vi "Draw circle.vi"(8 "error in (no error)":errorcluster, 10 "Detail in":T1, 11 "Image in":T2) -> (0 "error out":errorcluster, 3 "Image out":T2)   [LabVIEW 2019]
uses:
  <vilib>/vision/Image Controls.llb/IMAQ Image.ctl
  <vilib>/vision/NI_Vision_Development_Module.lvlib
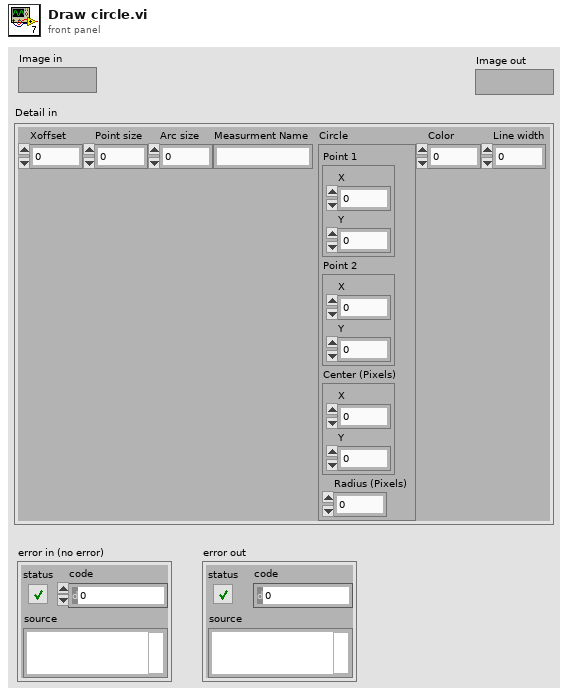
[diagram p1: front panel]
types:
  T1 = cluster{"Xoffset":i32, "Point size":dbl, "Arc size":dbl, "Measurment Name":string, "Circle":cluster{"Point 1":cluster{"X":sgl, "Y":sgl}, "Point 2":cluster{"X":sgl, "Y":sgl}, "Center (Pixels)":cluster{"X":sgl, "Y":sgl}, "Radius (Pixels)":dbl}, "Color":u32, "Line width":i32}
  T2 = typedef "IMAQ Image.ctl" = refnum<image>
  T3 = cluster{"Point 1":cluster{"X":sgl, "Y":sgl}, "Point 2":cluster{"X":sgl, "Y":sgl}, "Center (Pixels)":cluster{"X":sgl, "Y":sgl}, "Radius (Pixels)":dbl}
  T4 = cluster{"Left":i32, "Top":i32, "Right":i32, "Bottom":i32}
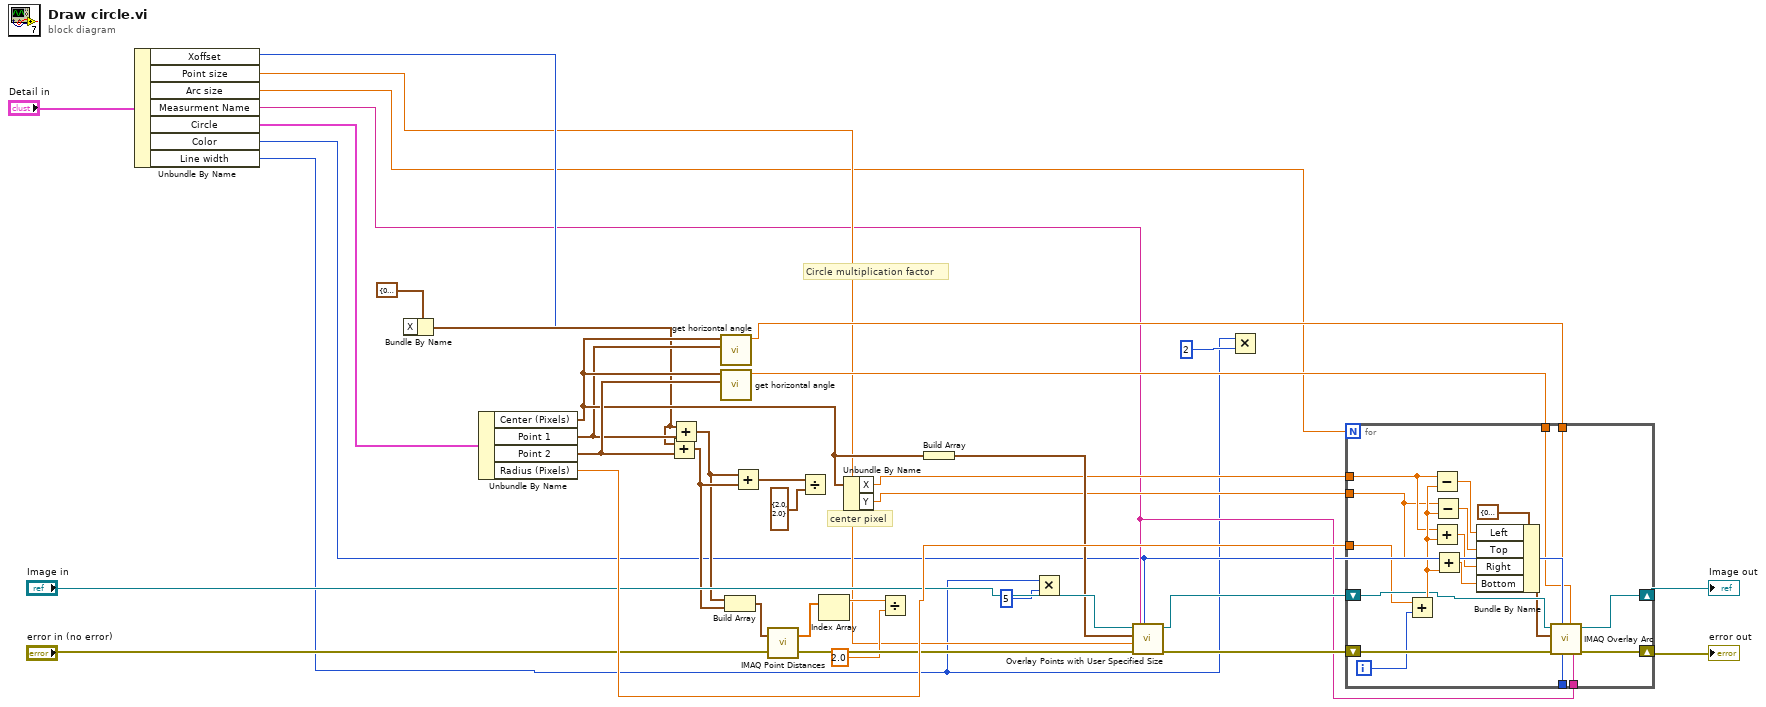
[diagram p0: block diagram]
diagram:
  # "Circle multiplication factor"
  # "center pixel"
  n1 = Unbundle By Name("Detail in") -> ("Xoffset"=w7:i32, "Point size"=w6:dbl, "Arc size"=w5:dbl, "Measurment Name"=w4:string, "Circle"=w3:T3, "Color"=w2:u32, "Line width"=w1:i32)
  n2 = Bundle By Name(cluster=cluster{"X":sgl, "Y":sgl} {"X"=0.0, "Y"=0.0} ("x"), "X"=w7) -> (w20:cluster{"X":sgl, "Y":sgl})
  n3 = Unbundle By Name(w3) -> ("Center (Pixels)"=w33:cluster{"X":sgl, "Y":sgl}, "Point 1"=w32:cluster{"X":sgl, "Y":sgl}, "Point 2"=w34:cluster{"X":sgl, "Y":sgl}, "Radius (Pixels)"=w31:dbl)
  n4 = Add(x=w20, y=w34) -> (x+y=w12:cluster{"X":sgl, "Y":sgl})
  n5 = Add(x=w20, y=w32) -> (x+y=w11:cluster{"X":sgl, "Y":sgl})
  n6 = call "get horizontal angle.vi"("Point 2"=w32, "Point 1"=w33) -> ("Angle w.r.t horizontal\n(in degrees)"=w35:sgl)  [unwired: 9 in]
  n7 = call "get horizontal angle.vi"("Point 2"=w34, "Point 1"=w33) -> ("Angle w.r.t horizontal\n(in degrees)"=w36:sgl)  [unwired: 9 in]
  n8 = Build Array(w11, w12) -> (w13:cluster{"X":sgl, "Y":sgl}[])
  n9 = Add(x=w11, y=w12) -> (x+y=w9:cluster{"X":sgl, "Y":sgl})
  n10 = call "IMAQ Point Distances"("Points"=w13, "error in (no error)"="error in (no error)") -> ("Distances"=w14:sgl[], "error out"=w26:errorcluster)  [unwired: 3 in]
  n11 = Divide(x=w9, y=cluster{"X":sgl, "Y":sgl} {"X"=2.0, "Y"=2.0}) -> ()  [unwired: 1 out]
  n12 = Index Array(array=w14) -> (element=w15:sgl)  [unwired: 1 in]
  n13 = Unbundle By Name(w33) -> ("X"=w21:sgl, "Y"=w22:sgl)
  n14 = Divide(x=w15, y=sgl 2.0) -> ()  [unwired: 1 out]
  n15 = Build Array(w33) -> (w28:cluster{"X":sgl, "Y":sgl}[])
  n16 = Multiply(x=w1, y=u32 5 ("Point Diameter (5)")) -> ()  [unwired: 1 out]
  n17 = call "Overlay Points with User Specified Size.vi"("Color"=w2, "Group"=w4, "error in"=w26, "Point Diameter (5)"=w6, "Points"=w28, "Image In"="Image in") -> ("error out"=w27:errorcluster, "Image Out"=w30:T2)  [unwired: 4 in]
  n18 = Multiply(x=w1, y=2) -> ()  [unwired: 1 out]
  n19 = for {
    N: w5 -> [_]
    shift-right: [w41] -> w18
    shift-left: w27 -> [w49]
    tunnel: w21 -> [w48]
    tunnel: w22 -> [w47]
    shift-right: [w46] -> w25
    shift-left: w30 -> [w45]
    tunnel: w31 -> [w43]
    tunnel: w2 -> [w42]
    tunnel: w35 -> [w39]
    tunnel: w36 -> [w38]
    tunnel: w4 -> [w37]
    i -> [w40]
    n20 = Add(x=w43, y=w40) -> (x+y=w50:dbl)
    n21 = Subtract(x=w48, y=w50) -> (x-y=w54:dbl)
    n22 = Add(x=w48, y=w50) -> (x+y=w52:dbl)
    n23 = Subtract(x=w47, y=w50) -> (x-y=w53:dbl)
    n24 = Add(x=w47, y=w50) -> (x+y=w51:dbl)
    n25 = Bundle By Name(cluster=T4 {"Left"=0, "Top"=0, "Right"=0, "Bottom"=0} ("Bounding Rectangle"), "Left"=w54, "Top"=w53, "Right"=w52, "Bottom"=w51) -> (w44:T4)
    n26 = call "IMAQ Overlay Arc"("Group"=w37, "End Angle (degrees)"=w38, "Color"=w42, "Start Angle (degrees)"=w39, "error in (no error)"=w49, "Bounding Rectangle"=w44, "Image"=w45) -> ("error out"=w41:errorcluster, "Image Out"=w46:T2)  [unwired: 3 in]
  }
  "Image out" <- w25
  "error out" <- w18
